vi "Read Minimum Energy.vi"(8 "error in (no error)":errorcluster, 11 "Burrow in":refnum<class "Burrow.lvclass">) -> (0 "error out":errorcluster, 2 "Minimum Energy":u64, 3 "Burrow out":refnum<class "Burrow.lvclass">)   [LabVIEW 2019, in "23.lvlib" / "Burrow.lvclass"]
uses:
  Burrow.lvclass
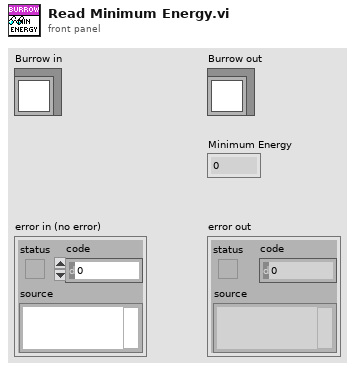
[diagram p1: front panel]
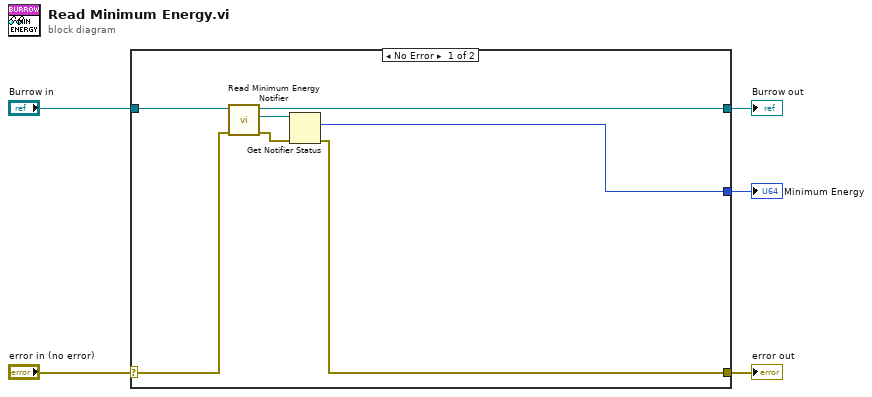
[diagram p0: block diagram]
diagram:
  n1 = case shown="No Error" "error in (no error)" {
    selector: "error in (no error)" -> [w12 w14]
    tunnel: [w7 w14] -> w4
    tunnel: [w11 w13] -> w2
    tunnel: "Burrow in" -> [w10 w13]
    tunnel: [w6 _] -> w1
    frame No Error {
      n2 = call-dynamic "Read Minimum Energy Notifier.vi"("error in (no error)"=w12, "Burrow in"=w10) -> ("error out"=w8:errorcluster, "Minimum Energy Notifier"=w9:refnum<notifier>, "Burrow out"=w11:refnum<class "Burrow.lvclass">)  [unwired: 7 in]
      n3 = Get Notifier Status(notifier=w9, error in (no error)=w8) -> (current notification=w6:u64, error out=w7:errorcluster)  [unwired: 3 out]
    }
    frame Error {
    }
  }
  "error out" <- w4
  "Burrow out" <- w2
  "Minimum Energy" <- w1
